vi "Read Multiple Waveforms.vi"(6 "Custom Source IDs":string[](array[string])=["", "Z2", "", "", "", "", "", "", "", ""], 8 "error in (no error)":errorcluster, 9 "Timeout (10000 ms)":u32=10000, 10 "Channels":u16[](array[ring])=[0, 1] items=["Channel 1", "Channel 2", "Channel 3", "Channel 4", "Memory 1", "Memory 2", "Memory 3", "Memory 4", "Function 1", "Function 2", "Function 3", "Function 4", "Function 5", "Function 6", "Function 7", "Function 8", "Other"], 11 "VISA resource name":refnum<visa-resource-name>) -> (0 "error out":errorcluster, 2 "Waveform Data":waveform(dbl)[](graph), 3 "VISA resource name out":refnum<visa-resource-name>)   [LabVIEW 2020, in "LeCroy Wave Series.lvlib"]
doc: "Initiates an acquisition on all channels that you enabled with the <B>Configure Channel</B> VI. The VI waits for the acquisition to complete and returns the waveform for the Source Channels you specified. If the oscilloscope did not complete the acquisition within the time period you specify with the Timeout parameter, the VI returns a time out error. A common cause for a timeout error is the acquisition was not triggered. For example, the trigger level is out of range of the waveform. \n\nNote: If your instrument does not support auto compensation for probe attenuation, you may need to adjust the scaling of the Waveform Data accordingly. This is handled automatically in the <B>Configure Channel</B> VI or can be done manually by multiplying the Waveform Data by the probe attenuation."
uses:
  LeCroy Wave Series.lvlib
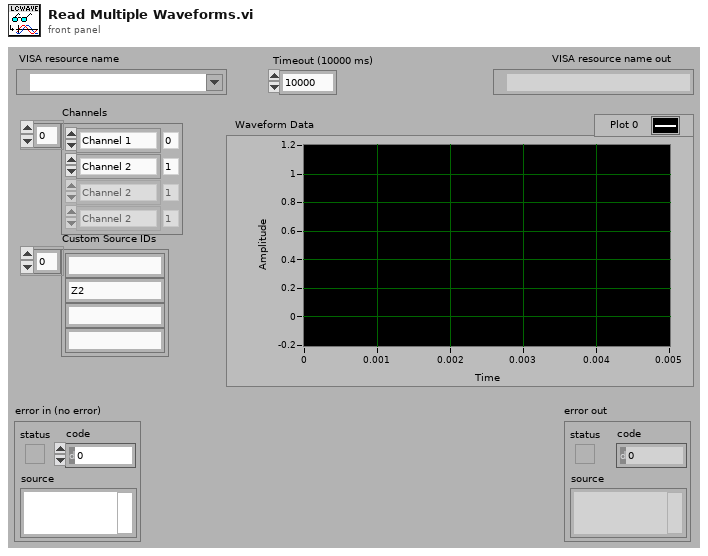
[diagram p1: front panel]
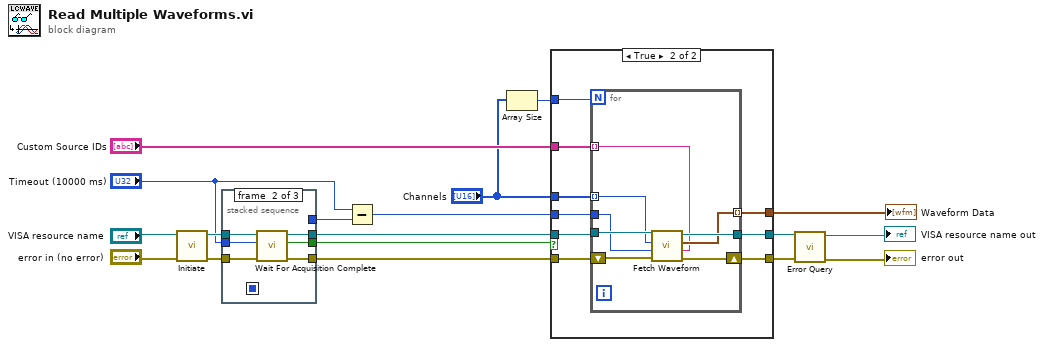
[diagram p0: block diagram]
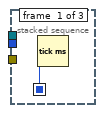
[diagram p2: hidden frame]
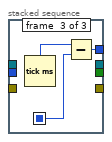
[diagram p3: hidden frame]
diagram:
  n1 = call "Initiate.vi"("error in (no error)"="error in (no error)", "VISA resource name"="VISA resource name") -> ("error out"=w10:errorcluster, "VISA resource name out"=w11:refnum<visa-resource-name>)  [unwired: 8 in]
  n2 = stacked-sequence {
    seq-local: [w19 _ _] -> [_ _ w27]
    tunnel: "Timeout (10000 ms)" -> [_ w25 _]
    tunnel: w11 -> [_ w23 _]
    tunnel: w10 -> [_ w21 _]
    tunnel: [_ w20 _] -> w13
    tunnel: [_ w22 _] -> w14
    tunnel: [_ _ w26] -> w15
    tunnel: [_ w24 _] -> w12
    frame #0 {
      n3 = Tick Count (ms)() -> (millisecond timer value=w19:u32)
    }
    frame #1 {
      n4 = call "Wait For Acquisition Complete.vi"("error in (no error)"=w21, "Timeout (10000 ms)"=w25, "VISA resource name"=w23) -> ("error out"=w20:errorcluster, "Complete"=w24:bool, "VISA resource name out"=w22:refnum<visa-resource-name>)  [unwired: 6 in]
    }
    frame #2 {
      n5 = Tick Count (ms)() -> (millisecond timer value=w28:u32)
      n6 = Subtract(x=w28, y=w27) -> (x-y=w26:u32)
    }
  }
  n7 = Subtract(x="Timeout (10000 ms)", y=w15) -> (x-y=w8:u32)
  n8 = Array Size(array="Channels") -> (size(s)=w1:i32)
  n9 = case shown="True" w12 {
    tunnel: [w30 w39] -> w7
    tunnel: [w29 w38] -> w6
    tunnel: [_ w37] -> w16
    tunnel: w14 -> [w30 w36]
    tunnel: w13 -> [w29 w35]
    tunnel: w8 -> [_ w34]
    tunnel: "Channels" -> [_ w33]
    tunnel: "Custom Source IDs" -> [_ w32]
    tunnel: w1 -> [_ w31]
    frame False {
    }
    frame True {
      n10 = for {
        N: w31 -> [_]
        tunnel: [w47] -> w39
        tunnel: w36 -> [w45]
        shift-right: [w46] -> w38
        shift-left: w35 -> [w44]
        tunnel: [w43] -> w37 mode=indexing
        tunnel: w34 -> [w41]
        tunnel: w33 -> [w42] mode=indexing
        tunnel: w32 -> [w40] mode=indexing
        n11 = call "Fetch Waveform.vi"("Custom Source ID"=w40, "error in (no error)"=w44, "Timeout (10000 ms)"=w41, "Source (0: Channel 1)"=w42, "VISA resource name"=w45) -> ("error out"=w46:errorcluster, "Waveform Graph"=w43:waveform(dbl), "VISA resource name out"=w47:refnum<visa-resource-name>)  [unwired: 4 in]
      }
    }
  }
  "Waveform Data" <- w16
  n12 = call "Error Query.vi"("error in (no error)"=w6, "VISA resource name"=w7) -> ("error out"=→"error out":errorcluster, "VISA resource name out"=→"VISA resource name out":refnum<visa-resource-name>)  [unwired: 6 in, 2 out]
